vi "close_refs.vi"(11 "Test Data in":T1) -> ()   [LabVIEW 2024, in "EncodingTester.lvlib"]
uses:
  EncodingTester.lvlib
  Tests/test_data--cluster.ctl
  Tests/packetized_data--cluster.ctl
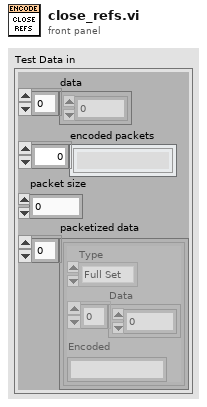
[diagram p1: front panel]
types:
  T1 = typedef "EncodingTester.lvlib/test_data--cluster.ctl" = cluster{"data":dbl[], "encoded packets":string[], "packet size":i32, "packetized data":T2[]}
  T2 = typedef "EncodingTester.lvlib/packetized_data--cluster.ctl" = cluster{"Type":enum16{"Full Set", "Last Set"}, "Data":dbl[], "Encoded":string}
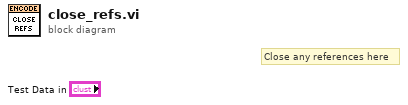
[diagram p0: block diagram]
diagram:
  # "Close any references here"
